vi "test_rethinkdb_all.vi"() -> (0 "error out":errorcluster, 3 "all_passed":bool)   [LabVIEW 2017]
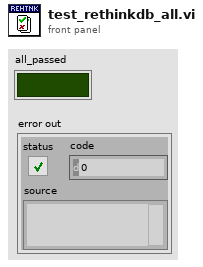
[diagram p1: front panel]
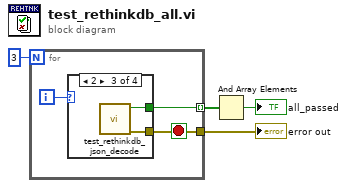
[diagram p0: block diagram]
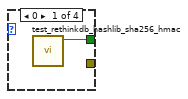
[diagram p2: hidden frame]
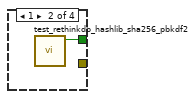
[diagram p3: hidden frame]
diagram:
  n1 = for {
    N: 3 -> [_]
    tunnel: [w6] -> w3 mode=indexing
    tunnel: [w5] -> w1
    i -> [w7]
    stop <- w5 stop-if-true
    n2 = case shown="2" w7 {
      tunnel: [w8 w9 w11 _] -> w6
      tunnel: [_ _ w10 _] -> w5
      frame 0 {
        n3 = call "test_rethinkdb_hashlib_sha256_hmac.vi"() -> ("all_passed"=w8:bool)  [unwired: 11 in]
      }
      frame 1 {
        n4 = call "test_rethinkdb_hashlib_sha256_pbkdf2.vi"() -> ("all_passed"=w9:bool)  [unwired: 11 in]
      }
      frame 2 {
        n5 = call "test_rethinkdb_json_decode.vi"() -> ("error out"=w10:errorcluster, "all_passed"=w11:bool)  [unwired: 10 in]
      }
      frame Default {
      }
    }
  }
  "error out" <- w1
  n6 = And Array Elements(Boolean array=w3) -> (logical AND=→"all_passed":bool)
